vi "AddRequest.vi"(5 "Reply Params Source":refnum<vi>, 7 "Request Params Source":refnum<vi>, 9 "Request Name":string, 10 "Module Name":string="TemplateModule", 11 "Module Ref":refnum<vi>) -> ()   [LabVIEW 2024, in "AddNewEvent.lvlib"]
uses:
  Event/AddNewEvent.lvlib
  templates/RequestTemplate.vi
  <vilib>/Utility/traverseref.llb/VI Scripting - Traverse.lvlib
  <vilib>/Utility/traverseref.llb/TRef TravTarget.ctl
  <vilib>/Utility/miscctls.llb/LVPositionTypeDef.ctl
  <vilib>/Utility/miscctls.llb/LVPoint32TypeDef.ctl
  <vilib>/_script/New VI Object TypeDefs/NewVIObject_LVRelativeDirectionTypeDef.ctl
  <vilib>/_script/New VI Object TypeDefs/NewVIObject_LVRelativePositionTypeDef.ctl
  Event/Templates/EHLRequest.vi
  <vilib>/event_ctls.llb/lveventtype.ctl
  Event/Templates/RequestMessageTemplate.ctl
  <vilib>/Utility/Data Type/NI_Data Type.lvlib
  <vilib>/Utility/miscctls.llb/LVPointTypeDef.ctl
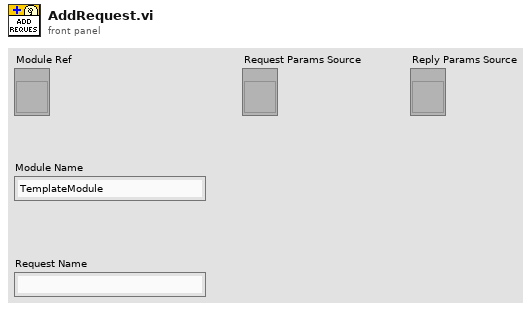
[diagram p1: front panel]
types:
  T1 = typedef "LVPositionTypeDef.ctl" = cluster{"Left":i32, "Top":i32}
  T2 = typedef "lveventtype.ctl" = enum32{"Null", "Timeout", "Annotation Menu Selection", "Annotation Menu Selection?", "App Instance Close", "App Instance Close?", "Autoscale Range Change", "Bookmark Info Change", "Cell Edit", "Cell Edit?", "Cursor Grab", "Cursor Grab?", "Cursor Menu Selection", "Cursor Menu Selection?", "Cursor Move", "Cursor Release", "Data Change", "Direction Change", "Display State Change", "Drag Ended", "Drag Enter", "Drag Leave", "Drag Over", "Drag Source Update", "Drag Starting", "Drag Starting?", "Drop", "Exec State Change", "Key Down", "Key Down?", "Key Repeat", "Key Repeat?", "Key Up", "Listbox Double Click", "Menu Activation?", "Menu Selection (App)", "Menu Selection? (App)", "Menu Selection (User)", "Mouse Down", "Mouse Down?", "Mouse Enter", "Mouse Leave", "Mouse Move", "Mouse Up", "Mouse Wheel", "NI Security User Change (App)", "Pane Size", "Panel Close", "Panel Close?", "Panel Resize", "Plot Attribute Change", "Scale Range Change", "Shortcut Menu Activation?", "Shortcut Menu Selection (App)", "Shortcut Menu Selection? (App)", "Shortcut Menu Selection (User)", "Tree Double Click", "Tree Drag", "Tree Drag?", "Tree Drop", "Tree Drop?", "Tree Item Close", "Tree Item Close?", "Tree Item Open", "Tree Item Open?", "User Event", "Value Change"}
  T3 = cluster{"Event Type":T2, "Reference":refnum<vi>, "Limit (-1=none)":i32, "Lock Panel?":bool}
  T4 = typedef "LVPointTypeDef.ctl" = cluster{"Horizontal":i16, "Vertical":i16}
  T5 = typedef "TRef TravTarget.ctl" = enum16{"FP", "BD", "Other"}
  T6 = enum32{"invalid VI type", "Standard VI", "Control VI", "Global VI", "Polymorphic VI", "Configuration VI", "SubSystem", "Facade VI", "Method VI", "Statechart Diagram VI"}
  T7 = cluster{"Event Type":T2, "Event Registration Index":i32}
  T8 = typedef "NewVIObject_LVRelativePositionTypeDef.ctl" = cluster{"Refnum":refnum<vi>, "Relative Direction":T9, "Point32":T10}
  T9 = typedef "NewVIObject_LVRelativeDirectionTypeDef.ctl" = enum32{"Right", "Left", "Top", "Bottom", "Top Right", "Top Left", "Bottom Right", "Bottom Left"}
  T10 = typedef "LVPoint32TypeDef.ctl" = cluster{"Horizontal":i32, "Vertical":i32}
  T11 = cluster{"Event Type":T2, "Event Registration Index":i32}[]
  T12 = cluster{"Event Type":T2, "Reference":refnum<vi>, "Limit (-1=none)":i32, "Lock Panel?":bool}[]
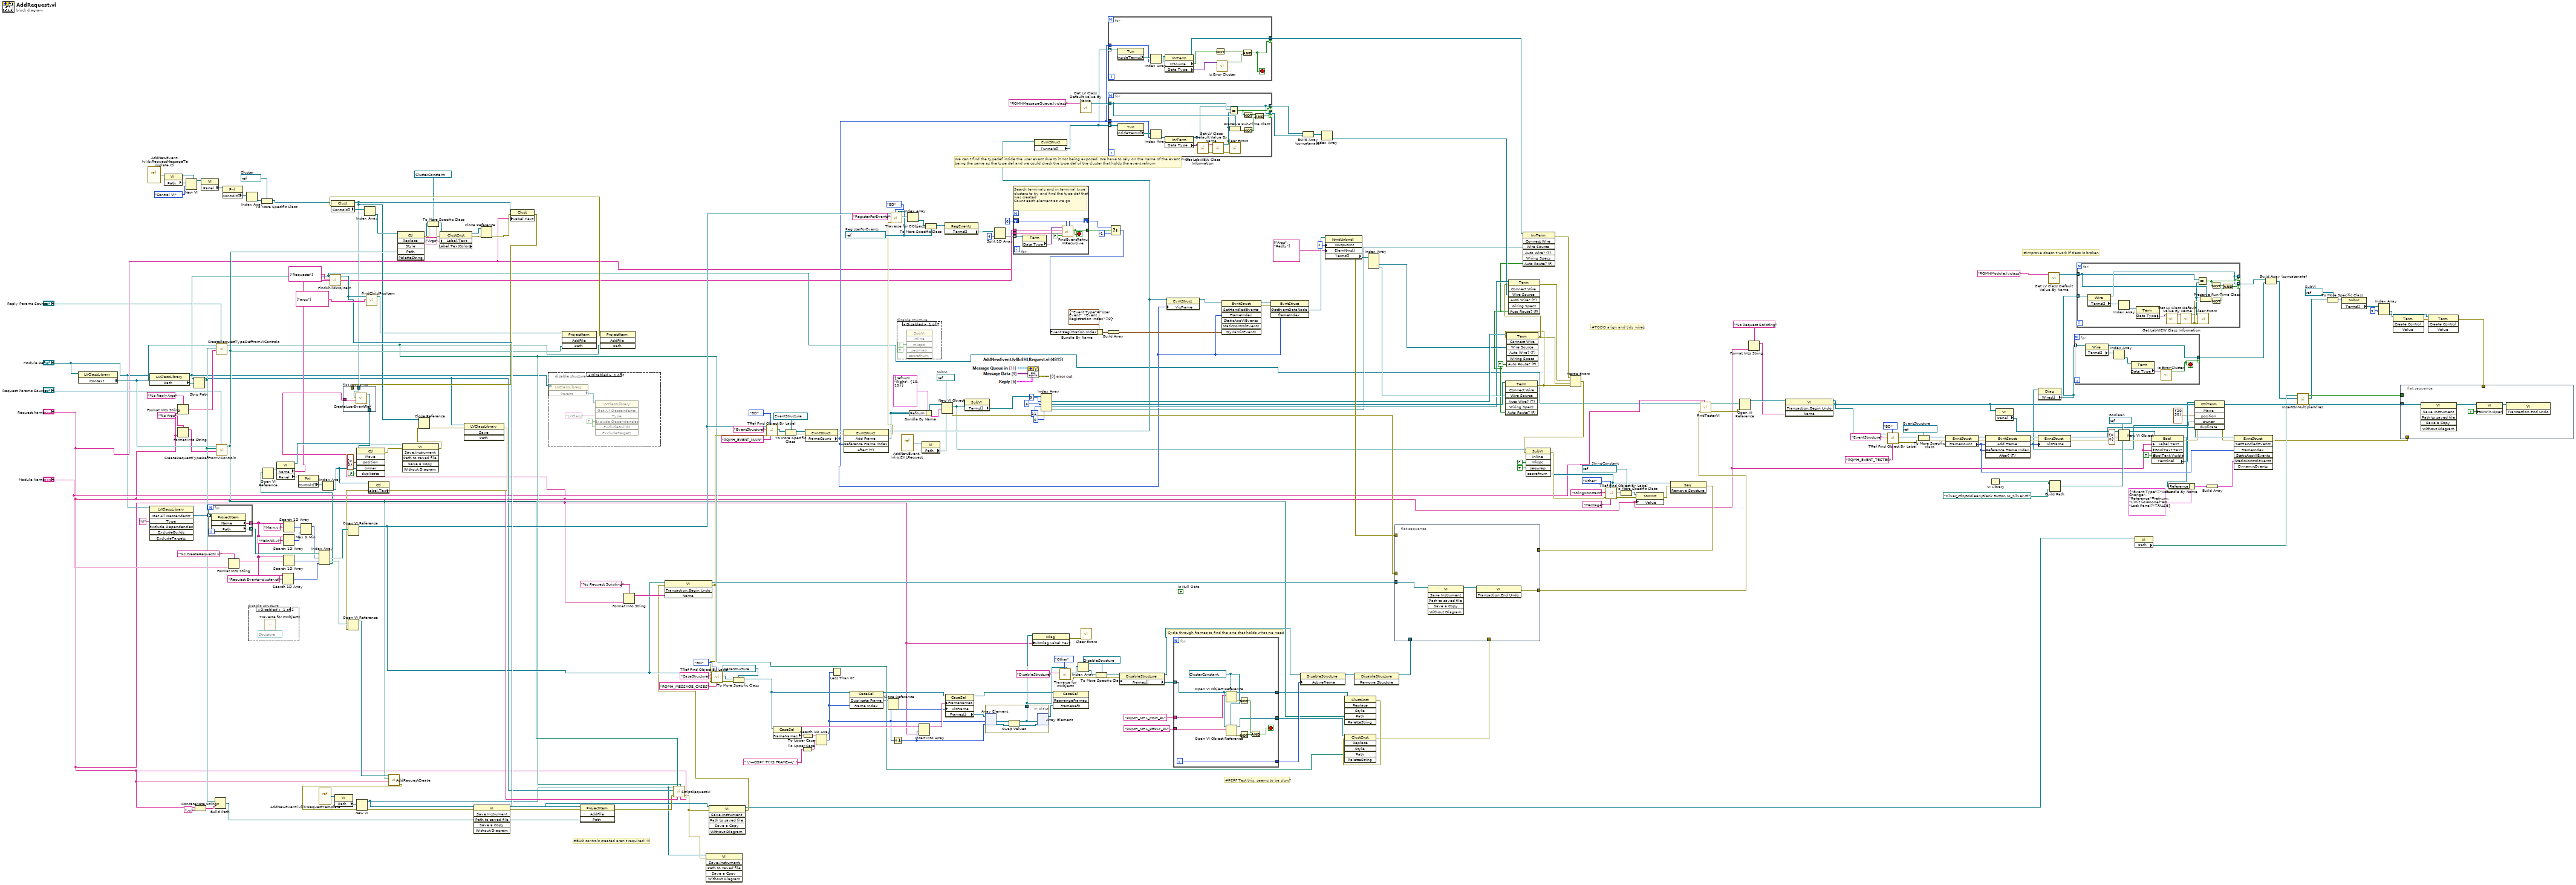
[diagram p0: block diagram]
diagram:
  w14 = refnum<vi> refnum  # SubVI
  w41 = refnum<vi> refnum  # Boolean
  w58 = refnum<vi> refnum  # EventStructure
  w82 = refnum<vi> refnum  # StringConstant
  w93 = TRUE ("Auto Route? (F)")
  w139 = refnum<vi> refnum  # Cluster
  w170 = refnum<vi> refnum  # RegisterForEvents
  w200 = refnum<vi> refnum  # SubVI
  (unwired) FALSE  # Is Null Data
  # "#BUG controls created aren't required!!!!!"
  # "#Improve doesn't work if class is broken"
  # "#TODO align and tidy wires"
  # "We can't find the typedef inside the user event due to it not being exposed. We have to rely on the name of the event num\nbeing the same as the type def and we could check the type def of the cluster that holds the event refnum"
  # "#PERF Test this, seems to be slow?"
  # "Cycle through frames to find the one that holds what we need"
  n1 = property class="LVClassLibrary"(reference="Module Ref") -> ("Context"=w213:refnum<vi>)  [unwired: 1 in, 2 out]
  n2 = vi-ref "AddNewEvent.lvlib:RequestMessageTemplate.ctl"() -> (w147:refnum<vi>)
  n3 = property class="LVClassLibrary"(reference="Module Ref") -> (reference out=w68:refnum<vi>, "Path"=w277:path)  [unwired: 1 in, 1 out]
  n4 = invoke class="LVClassLibrary" method="Get All Descendents"(reference="Module Ref", "Type"="VI") -> ("All Descendents"=w273:refnum<vi>[])  [unwired: 5 in, 6 out]
  n5 = property class="VI"(reference=w147) -> (reference out=w140:refnum<vi>, "Path"=w146:path)  [unwired: 1 in, 1 out]
  n6 = Format Into String(format string="%s ReplyArgs", "Request Name") -> (resulting string=w211:string)  [unwired: 2 in, 1 out]
  n7 = Format Into String(format string="%s Args", "Request Name") -> (resulting string=w208:string)  [unwired: 2 in, 1 out]
  n8 = New VI(5:w140, 9:T6."Control VI" ("vi type (standard vi)"), 10:w146) -> (3:w142:refnum<vi>)  [unwired: 4 in, 1 out]
  n9 = Strip Path(path=w277) -> (stripped path=w212:path)  [unwired: 1 out]
  n10 = Concatenate Strings("Request Name", ".vi" ("string")) -> (w247:string)
  n11 = property class="VI"(reference=w142) -> ("Panel"=w144:refnum<vi>)  [unwired: 1 in, 2 out]
  n12 = for {
    tunnel: w273 -> [w280] mode=indexing
    tunnel: [w279] -> w259 mode=indexing
    tunnel: [w278] -> w268 mode=indexing
    n13 = property class="ProjectItem"(reference=w280) -> ("Name"=w279:string, "Path"=w278:path)  [unwired: 1 in, 2 out]
  }
  n14 = Build Path(base path=w212, name or relative path=w247) -> (appended path=w246:path)
  n15 = call "CreateRequestTypeDefFromVIControls.vi"("VI Refnum"="Reply Params Source", "Control Name"=w211, "SaveFolderPath"=w212, "Application in"=w213) -> ("TypeDef Path"=w70:path)  [unwired: 6 in, 1 out]
  n16 = call "CreateRequestTypeDefFromVIControls.vi"("VI Refnum"="Request Params Source", "Control Name"=w208, "SaveFolderPath"=w212, "Application in"=w213) -> ("TypeDef Path"=w135:path)  [unwired: 6 in, 1 out]
  n17 = property class="Pnl"(reference=w144) -> ("Controls[]"=w143:refnum<vi>[])  [unwired: 1 in, 2 out]
  n18 = Format Into String(format string="%s.CreateRequests.vi" ("element"), "Module Name") -> (resulting string=w239:string)  [unwired: 2 in, 1 out]
  n19 = Index Array(array=w143) -> (element=w141:refnum<vi>)  [unwired: 1 in]
  n20 = disable-structure shown="Disabled" {
    frame Disabled {
      (unwired) refnum<vi> refnum ("Struct Refnum")
      n21 = call <vilib>:"Traverse for GObjects.vi"() -> ()  [unwired: 8 in, 4 out]
    }
    frame Enabled {
    }
  }
  n22 = To More Specific Class(target class=w139, reference=w141) -> (specific class reference=w138:refnum<vi>)  [unwired: 1 in, 1 out]
  n23 = Search 1D Array(1D array=w259, element="Request Events--cluster.ctl") -> (index of element=w258:i32)  [unwired: 1 in]
  n24 = Search 1D Array(1D array=w259, element=w239) -> (index of element=w267:i32)  [unwired: 1 in]
  n25 = Search 1D Array(1D array=w259, element="Main.vi") -> (index of element=w270:i32)  [unwired: 1 in]
  n26 = Search 1D Array(1D array=w259, element="MainNR.vi") -> (index of element=w269:i32)  [unwired: 1 in]
  n27 = Max & Min(x=w270, y=w269) -> (max(x,y)=w266:i32)  [unwired: 1 out]
  n28 = vi-ref "AddNewEvent.lvlib:RequestTemplate.vi"() -> (w276:refnum<vi>)
  n29 = Index Array(array=w268, index #1=w266, index #2=w267, index #3=w258) -> (element #1=w264:path, element #2=w265:path, element #3=w254:path)
  n30 = Open VI Reference(vi path=w254) -> (vi reference=w255:refnum<vi>)  [unwired: 5 in, 1 out]
  n31 = property class="VI"(reference=w255) -> (reference out=w205:refnum<vi>, "Name"=w157:string, "Panel"=w257:refnum<vi>)  [unwired: 1 in, 1 out]
  n32 = property class="Pnl"(reference=w257) -> ("Controls[]"=w256:refnum<vi>[])  [unwired: 1 in, 2 out]
  n33 = Index Array(array=w256) -> (element=w245:refnum<vi>)  [unwired: 1 in]
  n34 = call "FindChildProjItem.vi"("Level"=string[] ["Requests"], "ProjectItem in"=w68) -> ("Found or Orig"=w201:refnum<vi>)  [unwired: 8 in, 1 out]
  n35 = property class="VI"(reference=w276) -> ("Path"=w275:path)  [unwired: 1 in, 2 out]
  n36 = flat-sequence {
    tunnel: [w283] -> w251
    tunnel: "Request Name" -> [w282]
    tunnel: w131 -> [w281]
    tunnel: w129 -> [_]
    frame #0 {
      n37 = call "CreateUserEventRef.vi"("Label.Text"=w282, "referenceToEventRef"=w281) -> ("UserEventCtlRef"=w283:refnum<vi>)  [unwired: 9 in]
    }
  }
  n38 = Open VI Reference(vi path=w264) -> (vi reference=w160:refnum<vi>)  [unwired: 5 in, 1 out]
  n39 = invoke class="Ctl" method="Move"(reference=w251, "position"=T1 {"Left"=0, "Top"=0}, "owner"=w245, "duplicate"=FALSE ("Duplicate? (F)")) -> (error out=w207:errorcluster)  [unwired: 2 in, 5 out]
  n40 = call "FindChildProjItem.vi"("Level"=string[] ["args"], "ProjectItem in"=w201) -> ("Found or Orig"=w120:refnum<vi>)  [unwired: 8 in, 1 out]
  n41 = property class="Ctl"(reference=w245) -> ("Label.Text"=w244:string)  [unwired: 1 in, 2 out]
  n42 = invoke class="VI" method="Save.Instrument"(reference=w205, error in=w207) -> (error out=w206:errorcluster)  [unwired: 4 in, 5 out]
  n43 = disable-structure shown="Disabled" {
    disable-tunnel: w68 -> [w287 _]
    frame Disabled {
      w285 = TRUE ("ExcludeDependencies")
      n44 = property class="LVClassLibrary"(reference=w287) -> ("Parent"=w286:refnum<vi>)  [unwired: 1 in, 2 out]
      n45 = invoke class="LVClassLibrary" method="Get All Descendents"(reference=w286, "Type"="LVClass", "Exclude Dependencies"=w285, "ExcludeBuilds"=w285) -> ()  [unwired: 3 in, 7 out]
    }
    frame Enabled {
    }
  }
  n46 = invoke class="ProjectItem" method="AddFile"(reference=w120, "Path"=w135) -> (reference out=w121:refnum<vi>, error out=w204:errorcluster)  [unwired: 2 in, 2 out]
  n47 = property class="Clust"(reference=w138, error in=w204) -> (reference out=w131:refnum<vi>, "Controls[]"=w137:refnum<vi>[])  [unwired: 1 out]
  n48 = Index Array(array=w137) -> (element=w136:refnum<vi>)  [unwired: 1 in]
  n49 = invoke class="Ctl" method="Replace"(reference=w136, "Path"=w135) -> (error out=w128:errorcluster, "Replace"=w126:refnum<vi>)  [unwired: 4 in, 4 out]
  n50 = Close Reference(reference=w131, error in (no error)=w206) -> (error out=w262:errorcluster)
  n51 = To More Specific Class(target class=refnum<vi> refnum ("ClustCnst Refnum"), reference=w126, error in=w128) -> (specific class reference=w124:refnum<vi>, error out=w127:errorcluster)
  n52 = property class="ClustCnst" props=["Label", "Text", "Label", "TextColors"](reference=w124, error in=w127, "Label.Text"="Args") -> (reference out=w133:refnum<vi>, error out=w132:errorcluster)  [unwired: 1 out]
  n53 = invoke class="LVClassLibrary" method="Save"(reference=w68, error in=w262) -> (error out=w253:errorcluster)  [unwired: 2 in, 3 out]
  n54 = Open VI Reference(vi path=w265, error in (no error)=w253) -> (vi reference=w263:refnum<vi>)  [unwired: 4 in, 1 out]
  n55 = call "AddRequestCreate.vi"("New Name"="Request Name", "TypeDefPath"=w135, "VI in"=w263) -> ("error out"=w149:errorcluster)  [unwired: 8 in]
  n56 = New VI(8:w149, 10:w275) -> (0:w250:errorcluster, 3:w2:refnum<vi>)  [unwired: 5 in]
  n57 = invoke class="VI" method="Save.Instrument"(reference=w2, error in=w250, "Path to saved file"=w246) -> (reference out=w48:refnum<vi>, error out=w249:errorcluster)  [unwired: 3 in, 4 out]
  n58 = Close Reference(reference=w133, error in (no error)=w132) -> (error out=w130:errorcluster)
  n59 = property class="Clust"(reference=w131, error in=w130, "Label.Text"="Request Name") -> (error out=w129:errorcluster)  [unwired: 1 out]
  n60 = invoke class="ProjectItem" method="AddFile"(reference=w201, error in=w249, "Path"=w246) -> (error out=w148:errorcluster)  [unwired: 1 in, 3 out]
  n61 = invoke class="ProjectItem" method="AddFile"(reference=w121, "Path"=w70) -> ()  [unwired: 2 in, 4 out]
  n62 = Format Into String(format string="%s Request Scripting", "Request Name") -> (resulting string=w178:string)  [unwired: 2 in, 1 out]
  n63 = call "ScriptRequestVI.vi"("Request Name"="Request Name", "REPLYTypeDef Path"=w70, "EventClusterName"=w244, "REQTypeDef Path"=w135, "error in (no error)"=w148, "Module Ref"=w68, "VI in"=w2) -> ("error out"=w1:errorcluster)  [unwired: 4 in]
  n64 = invoke class="VI" method="Save.Instrument"(reference=w2, error in=w1) -> ()  [unwired: 4 in, 6 out]
  n65 = invoke class="VI" method="Save.Instrument"(reference=w48, error in=w1) -> (reference out=w46:refnum<vi>, error out=w47:errorcluster)  [unwired: 4 in, 4 out]
  n66 = invoke class="VI" method="Transaction.Begin Undo"(reference=w160, error in=w47, "Name"=w178) -> (reference out=w177:refnum<vi>, error out=w159:errorcluster)  [unwired: 1 in, 2 out]
  n67 = call <vilib>:"TRef Find Object By Label.vi"("Label"="RQMH_MESSAGE_CASES", "Traverse Target"=TRef_TravTarget."BD", "error in (no error)"=w159, "Class Name"="CaseStructure", "VI Ref"=w160) -> ("error out"=w181:errorcluster, "Found Obj Ref"=w182:refnum<vi>)  [unwired: 3 in, 2 out]
  n68 = To More Specific Class(target class=refnum<vi> refnum ("CaseSel Refnum"), reference=w182, error in=w181) -> (specific class reference=w180:refnum<vi>)  [unwired: 1 out]
  n69 = call <vilib>:"TRef Find Object By Label.vi"("Label"="RQMH_EVENT_MAIN", "Traverse Target"=TRef_TravTarget."BD", "error in (no error)"=w159, "Class Name"="EventStructure", "VI Ref"=w160) -> ("error out"=w196:errorcluster, "Found Obj Ref"=w195:refnum<vi>)  [unwired: 3 in, 2 out]
  n70 = property class="CaseSel"(reference=w180) -> ("FrameNames"=w225:string[])  [unwired: 1 in, 2 out]
  n71 = To More Specific Class(target class=refnum<vi> refnum ("EvntStruct Refnum"), reference=w195, error in=w196) -> (specific class reference=w191:refnum<vi>, error out=w193:errorcluster)
  n72 = To Upper Case(1:" \"---COPY THIS FRAME---\" " ("key")) -> (0:w237:string)
  n73 = To Upper Case(1:w225) -> (0:w238:string[])
  n74 = property class="EvntStruct"(reference=w191, error in=w193) -> (reference out=w174:refnum<vi>, error out=w192:errorcluster, "FrameCount"=w97:i32)
  n75 = Search 1D Array(1D array=w238, element=w237) -> (index of element=w222:i32)  [unwired: 1 in]
  n76 = Less Than 0?(x=w222) -> ()  [unwired: 1 out]
  n77 = invoke class="EvntStruct" method="Add Frame"(reference=w174, error in=w192, "Reference Frame Index"=w97) -> (reference out=w107:refnum<vi>, error out=w158:errorcluster, "Add Frame"=w108:refnum<vi>)  [unwired: 2 in, 2 out]
  n78 = invoke class="CaseSel" method="Duplicate Frame"(reference=w180, "Frame Index"=w222) -> (reference out=w235:refnum<vi>, "Duplicate Frame"=w231:refnum<vi>)  [unwired: 2 in, 2 out]
  n79 = Close Reference(reference=w231) -> ()  [unwired: 1 in, 1 out]
  n80 = call <vilib>:"Traverse for GObjects.vi"("Other Refnum"=w170, "Traverse Target"=TRef_TravTarget."BD", "error in (no error)"=w158, "Class Name"="RegisterForEvents", "VI Refnum"=w160) -> ("References"=w171:refnum<vi>[])  [unwired: 3 in, 3 out]
  n81 = Increment(x=w222) -> (x+1=w223:i32)
  n82 = disable-structure shown="Disabled" {
    frame Disabled {
      n83 = invoke class="SubVI" method="Inline"("mkspc"=TRUE ("Make Space in Block Diagram"), "seqwrap"=TRUE ("Wrap in Sequence")) -> ()  [unwired: 4 in, 6 out]
    }
    frame Enabled {
    }
  }
  n84 = vi-ref "AddNewEvent.lvlib:EHLRequest.vi"() -> (w189:refnum<vi>)
  n85 = Index Array(array=w171) -> (element=w169:refnum<vi>)  [unwired: 1 in]
  n86 = Bundle By Name(cluster=T8 {"Refnum"=refnum, "Relative Direction"=enum."Right", "Point32"={"Horizontal"=10, "Vertical"=10}} ("Relative Position"), "Refnum"=w108) -> (w187:T8)
  n87 = Insert Into Array(array=w225, index=w223, new element="Request Name") -> (w224:string[])
  n88 = property class="VI"(reference=w189) -> ("Path"=w188:path)  [unwired: 1 in, 2 out]
  n89 = To More Specific Class(target class=w170, reference=w169) -> (specific class reference=w168:refnum<vi>)  [unwired: 1 in, 1 out]
  n90 = New VI Object(vi object class=w200, owner refnum=w108, position/next to=w187, 6:w188) -> (object refnum=w89:refnum<vi>, 0:w175:errorcluster)  [unwired: 4 in]
  n91 = property class="RegEvents"(reference=w168) -> ("Terms[]"=w167:refnum<vi>[])  [unwired: 1 in, 2 out]
  n92 = property class="CaseSel"(reference=w235, "FrameNames"=w224, "VisFrame"=w222) -> (reference out=w234:refnum<vi>, "Frames[]"=w233:refnum<vi>[])  [unwired: 1 in, 1 out]
  n93 = property class="SubVI"(reference=w89) -> ("Terms[]"=w116:refnum<vi>[])  [unwired: 1 in, 2 out]
  n94 = in-place {
    in-place-border: [w290] -> w226
    n95 = in-place-array #1(w233, w222, w223) -> (w293:refnum<vi>, w292:refnum<vi>)
    n96 = Swap Values(12:w293, 14:w292) -> (1:w290:refnum<vi>, 3:w291:refnum<vi>)  [unwired: 1 in]
    n97 = in-place-array #1(w290, w291) -> (w232:refnum<vi>[])  [unwired: 2 out]
  }
  n98 = Split 1D Array(array=w167, index=4) -> (second subarray=w165:refnum<vi>[])  [unwired: 1 out]
  n99 = for {
    tunnel: w165 -> [w301] mode=indexing
    tunnel: "Request Name" -> [w296]
    shift-right: [w300] -> w161
    shift-left: 0 -> [w299]
    tunnel: [w298] -> w163
    tunnel: w157 -> [w295]
    stop <- w298 stop-if-true
    # "Search terminals and in terminal type clusters to try and find the type def that was created\nCount each element as we go"
    n100 = property class="Term"(reference=w301) -> ("Data Type"=w297:variant)  [unwired: 1 in, 2 out]
    n101 = call "FindEventRefnumRecursive.vi"("count in"=w299, "InNamedTypedef?"=FALSE, "Event name"=w296, "Event holder typedef"=w295, "Data Type"=w297) -> ("Found?"=w298:bool, "count out"=w300:i32)  [unwired: 5 in]
  }
  n102 = property class="Diag"(reference=w226, "SubDiag Label.Text"="Request Name") -> (error out=w230:errorcluster)  [unwired: 1 in, 1 out]
  n103 = property class="EvntStruct"(reference=w107) -> ("Tunnels[]"=w96:refnum<vi>[])  [unwired: 1 in, 2 out]
  n104 = Index Array(array=w116, index #1=9 ("index"), index #2=6 ("index"), index #3=11 ("index"), index #4=0 ("index")) -> (element #1=w112:refnum<vi>, element #2=w111:refnum<vi>, element #3=w101:refnum<vi>, element #4=w94:refnum<vi>)
  n105 = invoke class="CaseSel" method="RearrangeFrames"(reference=w234, "FrameRefs"=w232) -> ()  [unwired: 2 in, 4 out]
  n106 = call <vilib>:"Traverse for GObjects.vi"("Other Refnum"=w226, "Traverse Target"=TRef_TravTarget."Other", "Class Name"="DisableStructure") -> ("error out"=w229:errorcluster, "References"=w228:refnum<vi>[])  [unwired: 5 in, 2 out]
  n107 = Index Array(array=w228) -> (element=w227:refnum<vi>)  [unwired: 1 in]
  n108 = call <vilib>:"Get LV Class Default Value By Name.vi"("class name"="RQMHMessageQueue.lvclass") -> ("object"=w105:refnum<class>)  [unwired: 9 in, 1 out]
  n109 = call <vilib>:"Clear Errors.vi"("error in (no error)"=w230) -> ()  [unwired: 5 in, 2 out]
  n110 = To More Specific Class(target class=refnum<vi> refnum ("DisableStructure Refnum"), reference=w227, error in=w229) -> (specific class reference=w221:refnum<vi>, error out=w220:errorcluster)
  n111 = for {
    tunnel: w96 -> [w311] mode=indexing
    tunnel: w97 -> [w308]
    tunnel: [w302] -> w95 if=w303
    stop <- w303 stop-if-true
    n112 = property class="Tun"(reference=w311) -> ("InsideTerms[]"=w310:refnum<vi>[])  [unwired: 1 in, 2 out]
    n113 = Index Array(array=w310, index=w308) -> (element=w309:refnum<vi>)
    n114 = property class="InrTerm"(reference=w309) -> (reference out=w302:refnum<vi>, "IsSource"=w305:bool, "Data Type"=w307:variant)  [unwired: 1 in, 1 out]
    n115 = Not(x=w305) -> (.not. x?=w304:bool)
    n116 = call <vilib>:"Is Error Cluster.vi"("variant"=w307) -> ("is error cluster?"=w306:bool)  [unwired: 9 in, 1 out]
    n117 = And(x=w304, y=w306) -> (x .and. y?=w303:bool)
  }
  n118 = for {
    tunnel: w96 -> [w327] mode=indexing
    tunnel: w105 -> [w321]
    tunnel: [w312] -> w104 mode=indexing if=w319
    tunnel: [w312] -> w103 mode=indexing if=w316
    tunnel: w97 -> [w315]
    n119 = property class="Tun"(reference=w327) -> ("InsideTerms[]"=w326:refnum<vi>[])  [unwired: 1 in, 2 out]
    n120 = Index Array(array=w326, index=w315) -> (element=w325:refnum<vi>)
    n121 = property class="InrTerm"(reference=w325) -> (reference out=w312:refnum<vi>, "Data Type"=w324:variant)  [unwired: 1 in, 1 out]
    n122 = call <vilib>:"Get LabVIEW Class Information.vi"("variant"=w324) -> ("error out"=w314:errorcluster, "LabVIEW class file name"=w323:string)  [unwired: 8 in, 1 out]
    n123 = call <vilib>:"Get LV Class Default Value By Name.vi"("error in (no error)"=w314, "class name"=w323) -> ("error out"=w313:errorcluster, "object"=w320:refnum<class>)  [unwired: 8 in]
    n124 = Equal?(x=w321, y=w320) -> (x = y?=w319:bool)
    n125 = Preserve Run-Time Class(object in=w320, 2:w321) -> (error out=w322:errorcluster)  [unwired: 1 in, 1 out]
    n126 = call <vilib>:"Clear Errors.vi"("error in (no error)"=w313) -> ()  [unwired: 5 in, 2 out]
    n127 = Not(x=w319) -> (.not. x?=w317:bool)
    n128 = Not(x=w322) -> (.not. x?=w318:bool)
    n129 = And(x=w317, y=w318) -> (x .and. y?=w316:bool)
  }
  n130 = Select(t=w161, s=w163, f=-1) -> (s? t:f=w150:i32)
  n131 = Bundle By Name(cluster=T7 {"Event Type"=enum."User Event", "Event Registration Index"=0} ("Dynamic Events"), "Event Registration Index"=w150) -> (w156:T7)
  n132 = Build Array(w156) -> (w154:T11)
  n133 = property class="DisableStructure"(reference=w221, error in=w220) -> (reference out=w216:refnum<vi>, "Frames[]"=w219:refnum<vi>[])  [unwired: 1 out]
  n134 = property class="EvntStruct"(reference=w107, "VisFrame"=w97) -> (reference out=w123:refnum<vi>)  [unwired: 1 in, 1 out]
  n135 = for {
    tunnel: w219 -> [w339] mode=indexing
    tunnel: "RQMH_MHL_REPLY_PL" -> [w337]
    tunnel: "RQMH_MHL_MSG_PL" -> [w336]
    tunnel: [w335] -> w214
    tunnel: [w334] -> w73
    tunnel: [w332] -> w215
    i -> [w332]
    stop <- w328 stop-if-true
    w333 = refnum<vi> refnum ("ClustCnst Refnum")
    n136 = Open VI Object Reference(7:w333, 10:w336, 11:w339) -> (0:w338:errorcluster, 3:w335:refnum<vi>)  [unwired: 1 in]
    n137 = Open VI Object Reference(7:w333, 10:w337, 11:w339) -> (0:w331:errorcluster, 3:w334:refnum<vi>)  [unwired: 1 in]
    n138 = Not(x=w338) -> (.not. x?=w329:bool)
    n139 = Not(x=w331) -> (.not. x?=w330:bool)
    n140 = And(x=w329, y=w330) -> (x .and. y?=w328:bool)
  }
  n141 = invoke class="EvntStruct" method="SetHandledEvents"(reference=w123, "FrameIndex"=w97, "DynamicEvents"=w154) -> (reference out=w152:refnum<vi>, error out=w153:errorcluster)  [unwired: 4 in, 5 out]
  n142 = invoke class="EvntStruct" method="GetEventDataNode"(reference=w152, error in=w153, "frameIndex"=w97) -> ("GetEventDataNode"=w151:refnum<vi>)  [unwired: 1 in, 3 out]
  n143 = property class="DisableStructure"(reference=w216, "ActiveFrame"=w215) -> (reference out=w176:refnum<vi>)  [unwired: 1 in, 1 out]
  n144 = Build Array (concatenate)(w104, w103) -> (w102:refnum<vi>[])
  n145 = Index Array(array=w102) -> (element=w100:refnum<vi>)  [unwired: 1 in]
  n146 = property class="NmdUnbndl"(reference=w151, "OutputCnt"=2 ("Output Count"), "ElemNms[]"=string[] ["Args", "Reply"] ("Element Names[]")) -> (error out=w122:errorcluster, "Terms[]"=w117:refnum<vi>[])  [unwired: 1 in, 1 out]
  n147 = invoke class="ClustCnst" method="Replace"(reference=w214, "Path"=w135) -> (error out=w72:errorcluster)  [unwired: 4 in, 5 out]
  n148 = invoke class="ClustCnst" method="Replace"(reference=w73, error in=w72, "Path"=w70) -> (error out=w71:errorcluster)  [unwired: 3 in, 5 out]
  n149 = invoke class="DisableStructure" method="Remove Structure"(reference=w176) -> (reference out=w74:refnum<vi>)  [unwired: 2 in, 2 out]
  n150 = Index Array(array=w117) -> (element #2=w110:refnum<vi>, element #3=w109:refnum<vi>)  [unwired: 3 in, 1 out]
  n151 = flat-sequence {
    tunnel: w177 -> [w342]
    tunnel: w74 -> [_]
    tunnel: w175 -> [_]
    tunnel: w122 -> [_]
    tunnel: w75 -> [_]
    tunnel: w71 -> [_]
    tunnel: [w341] -> w65
    frame #0 {
      n152 = invoke class="VI" method="Save.Instrument"(reference=w342) -> (reference out=w340:refnum<vi>)  [unwired: 5 in, 5 out]
      n153 = invoke class="VI" method="Transaction.End Undo"(reference=w340) -> (error out=w341:errorcluster)  [unwired: 2 in, 2 out]
    }
  }
  n154 = invoke class="Term" method="Connect Wire"(reference=w111, "Wire Source"=w109, "Auto Route? (F)"=w93) -> (error out=w90:errorcluster)  [unwired: 4 in, 6 out]
  n155 = invoke class="Term" method="Connect Wire"(reference=w112, error in=w90, "Wire Source"=w110, "Auto Route? (F)"=w93) -> (error out=w91:errorcluster)  [unwired: 3 in, 6 out]
  n156 = invoke class="Term" method="Connect Wire"(reference=w101, error in=w91, "Wire Source"=w100, "Auto Route? (F)"=w93) -> (error out=w99:errorcluster)  [unwired: 3 in, 6 out]
  n157 = invoke class="InrTerm" method="Connect Wire"(reference=w95, "Wire Source"=w94, "Auto Route? (F)"=w93) -> (error out=w92:errorcluster)  [unwired: 4 in, 6 out]
  n158 = Merge Errors(w92, w99, w91, w90) -> (w87:errorcluster)
  n159 = invoke class="SubVI" method="Inline"(reference=w89, error in=w87, "mkspc"=FALSE ("Make Space in Block Diagram"), "seqwrap"=TRUE ("Wrap in Sequence")) -> (error out=w79:errorcluster, "seqrefnum"=w77:refnum<vi>)  [unwired: 2 in, 4 out]
  n160 = call <vilib>:"TRef Find Object By Label.vi"("Other Refnum"=w77, "Label"="Message" ("name/order"), "Traverse Target"=TRef_TravTarget."Other", "error in (no error)"=w79, "Class Name"="StringConstant") -> ("error out"=w78:errorcluster, "Found Obj Ref"=w81:refnum<vi>)  [unwired: 3 in, 2 out]
  n161 = To More Specific Class(target class=w82, reference=w81) -> (specific class reference=w80:refnum<vi>)  [unwired: 1 in, 1 out]
  n162 = property class="StrCnst"(reference=w80, error in=w78, "Value"="Request Name") -> (error out=w76:errorcluster)  [unwired: 1 out]
  n163 = invoke class="Seq" method="Remove Structure"(reference=w77, error in=w76) -> (error out=w75:errorcluster)  [unwired: 1 in, 2 out]
  n164 = call "FindTesterVI.vi"("Module Name"="Module Name", "error in (no error)"=w65, "module ref"=w68) -> ("error out"=w66:errorcluster, "TesterPath"=w67:path)  [unwired: 7 in]
  n165 = Open VI Reference(vi path=w67, error in (no error)=w66) -> (vi reference=w64:refnum<vi>)  [unwired: 4 in, 1 out]
  n166 = Format Into String(format string="%s Request Scripting" ("Name"), "Request Name") -> (resulting string=w59:string)  [unwired: 2 in, 1 out]
  n167 = invoke class="VI" method="Transaction.Begin Undo"(reference=w64, "Name"=w59) -> (reference out=w40:refnum<vi>)  [unwired: 2 in, 3 out]
  n168 = call <vilib>:"TRef Find Object By Label.vi"("Label"="RQMH_EVENT_TESTER", "Traverse Target"=TRef_TravTarget."BD", "Class Name"="EventStructure", "VI Ref"=w40) -> ("error out"=w52:errorcluster, "Found Obj Ref"=w56:refnum<vi>)  [unwired: 4 in, 2 out]
  n169 = To More Specific Class(target class=w58, reference=w56, error in=w52) -> (specific class reference=w57:refnum<vi>, error out=w53:errorcluster)
  n170 = property class="EvntStruct"(reference=w57, error in=w53) -> (reference out=w55:refnum<vi>, error out=w54:errorcluster, "FrameCount"=w22:i32)
  n171 = invoke class="EvntStruct" method="Add Frame"(reference=w55, error in=w54, "Reference Frame Index"=w22) -> (reference out=w51:refnum<vi>, error out=w50:errorcluster, "Add Frame"=w18:refnum<vi>)  [unwired: 2 in, 2 out]
  n172 = VI Library() -> (path=w44:path)
  n173 = property class="VI"(reference=w40) -> ("Panel"=w39:refnum<vi>)  [unwired: 1 in, 2 out]
  n174 = property class="EvntStruct"(reference=w51, error in=w50, "VisFrame"=w22) -> (reference out=w35:refnum<vi>, error out=w45:errorcluster)
  n175 = property class="Diag"(reference=w18) -> ("Wires[]"=w21:refnum<vi>[])  [unwired: 1 in, 2 out]
  n176 = call <vilib>:"Get LV Class Default Value By Name.vi"("class name"="RQMHModule.lvclass") -> ("object"=w24:refnum<class>)  [unwired: 9 in, 1 out]
  n177 = Build Path(base path=w44, name or relative path=path "silver_ctls/Boolean/Blank Button NI_Silver.ctl") -> (appended path=w42:path)
  n178 = for {
    tunnel: w21 -> [w348] mode=indexing
    tunnel: [w344] -> w49 if=w343
    stop <- w343 stop-if-true
    n179 = property class="Wire"(reference=w348) -> (reference out=w344:refnum<vi>, "Terms[]"=w347:refnum<vi>[])  [unwired: 1 in, 1 out]
    n180 = Index Array(array=w347) -> (element=w346:refnum<vi>)  [unwired: 1 in]
    n181 = property class="Term"(reference=w346) -> ("Data Type"=w345:variant)  [unwired: 1 in, 2 out]
    n182 = call <vilib>:"Is Error Cluster.vi"("variant"=w345) -> ("is error cluster?"=w343:bool)  [unwired: 9 in, 1 out]
  }
  n183 = for {
    tunnel: w21 -> [w363] mode=indexing
    tunnel: w24 -> [w350]
    tunnel: [w353] -> _ mode=indexing if=w358
    tunnel: [w353] -> w20 mode=indexing if=w355
    n184 = property class="Wire"(reference=w363) -> (reference out=w353:refnum<vi>, "Terms[]"=w362:refnum<vi>[])  [unwired: 1 in, 1 out]
    n185 = Index Array(array=w362) -> (element=w361:refnum<vi>)  [unwired: 1 in]
    n186 = property class="Term"(reference=w361) -> ("Data Type"=w352:variant)  [unwired: 1 in, 2 out]
    n187 = call <vilib>:"Get LabVIEW Class Information.vi"("variant"=w352) -> ("error out"=w354:errorcluster, "LabVIEW class file name"=w360:string)  [unwired: 8 in, 1 out]
    n188 = call <vilib>:"Get LV Class Default Value By Name.vi"("error in (no error)"=w354, "class name"=w360) -> ("error out"=w351:errorcluster, "object"=w349:refnum<class>)  [unwired: 8 in]
    n189 = Equal?(x=w350, y=w349) -> (x = y?=w358:bool)
    n190 = call <vilib>:"Clear Errors.vi"("error in (no error)"=w351) -> ()  [unwired: 5 in, 2 out]
    n191 = Preserve Run-Time Class(object in=w349, error in=w351, 2:w350) -> (error out=w359:errorcluster)  [unwired: 1 out]
    n192 = Not(x=w358) -> (.not. x?=w356:bool)
    n193 = Not(x=w359) -> (.not. x?=w357:bool)
    n194 = And(x=w356, y=w357) -> (x .and. y?=w355:bool)
  }
  n195 = New VI Object(vi object class=w41, owner refnum=w39, position/next to=T4 {"Horizontal"=0, "Vertical"=0} ("location"), 6:w42, 8:w45) -> (object refnum=w37:refnum<vi>, 0:w36:errorcluster)  [unwired: 3 in]
  n196 = property class="VI"(reference=w46) -> ("Path"=w23:path)  [unwired: 1 in, 2 out]
  n197 = property class="Bool"(reference=w37, error in=w36, "Label.Text"="Request Name", "BoolText.Text"="Request Name", "BoolText.Visible"=TRUE ("Boolean Text.Visible")) -> (reference out=w31:refnum<vi>, error out=w29:errorcluster, "Terminal"=w27:refnum<vi>)
  n198 = Bundle By Name(cluster=T3 {"Event Type"=enum."Value Change", "Reference"=refnum, "Limit (-1=none)"=0, "Lock Panel?"=FALSE} ("Static Control Events"), "Reference"=w31) -> (w33:T3)
  n199 = invoke class="CtrlTerm" method="Move"(reference=w27, error in=w29, "position"=T1 {"Left"=20, "Top"=30}, "owner"=w18) -> (error out=w28:errorcluster)  [unwired: 2 in, 5 out]
  n200 = Build Array(w33) -> (w32:T12)
  n201 = invoke class="EvntStruct" method="SetHandledEvents"(reference=w35, error in=w28, "FrameIndex"=w22, "StaticControlEvents"=w32) -> (error out=w17:errorcluster)  [unwired: 3 in, 6 out]
  n202 = Build Array (concatenate)(w20, w49) -> (w19:refnum<vi>[])
  n203 = call "InsertOnMultipleWires.vi"("Wire Array"=w19, "To Insert"=w23) -> ("Inserted"=w15:refnum<vi>, "Done?"=w16:bool)  [unwired: 8 in]
  n204 = To More Specific Class(target class=w14, reference=w15) -> (specific class reference=w13:refnum<vi>)  [unwired: 1 in, 1 out]
  n205 = property class="SubVI"(reference=w13) -> ("Terms[]"=w12:refnum<vi>[])  [unwired: 1 in, 2 out]
  n206 = Index Array(array=w12, index #1=9 ("index")) -> (element #1=w10:refnum<vi>, element #2=w9:refnum<vi>)  [unwired: 1 in]
  n207 = invoke class="Term" method="Create Control"(reference=w10) -> (error out=w8:errorcluster)  [unwired: 3 in, 3 out]
  n208 = flat-sequence {
    tunnel: w40 -> [w364]
    tunnel: w17 -> [_]
    tunnel: w16 -> [_]
    tunnel: w7 -> [_]
    frame #0 {
      n209 = invoke class="VI" method="Save.Instrument"(reference=w364) -> (reference out=w365:refnum<vi>)  [unwired: 5 in, 5 out]
      n210 = property class="VI"(reference=w365, "BDWin.Open"=TRUE ("Block Diagram Window:Open")) -> (reference out=w367:refnum<vi>)  [unwired: 1 in, 1 out]
      n211 = invoke class="VI" method="Transaction.End Undo"(reference=w367) -> ()  [unwired: 2 in, 3 out]
    }
  }
  n212 = invoke class="Term" method="Create Control"(reference=w9, error in=w8) -> (error out=w7:errorcluster)  [unwired: 2 in, 3 out]
